vi "sub_thresh_swing_subvi.vi"(0 "Path":path, 9 "NumPts":dbl=3.0, 11 "Row Start":dbl=20.0) -> (3 "Index":dbl, 4 "XY Graph":cluster{dbl[], dbl[]}[](graph), 12 "Table Control":string[][](table), 13 "Table Control 2":string[][](table), 15 "Sub Threshold Swing":dbl)   [LabVIEW 2011]
uses:
  <vilib>/Utility/file.llb/Read From Spreadsheet File (string).vi
  <vilib>/Analysis/NI_AALPro.lvlib
panel:
  out "Numeric":dbl
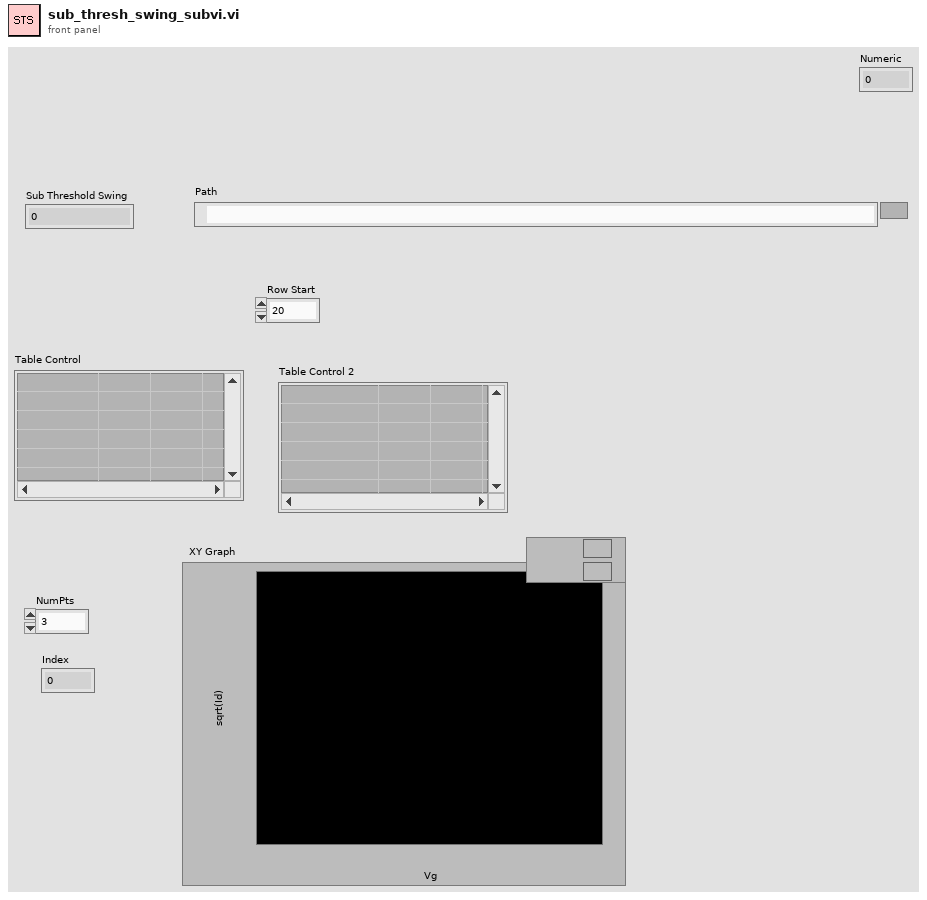
[diagram p1: front panel]
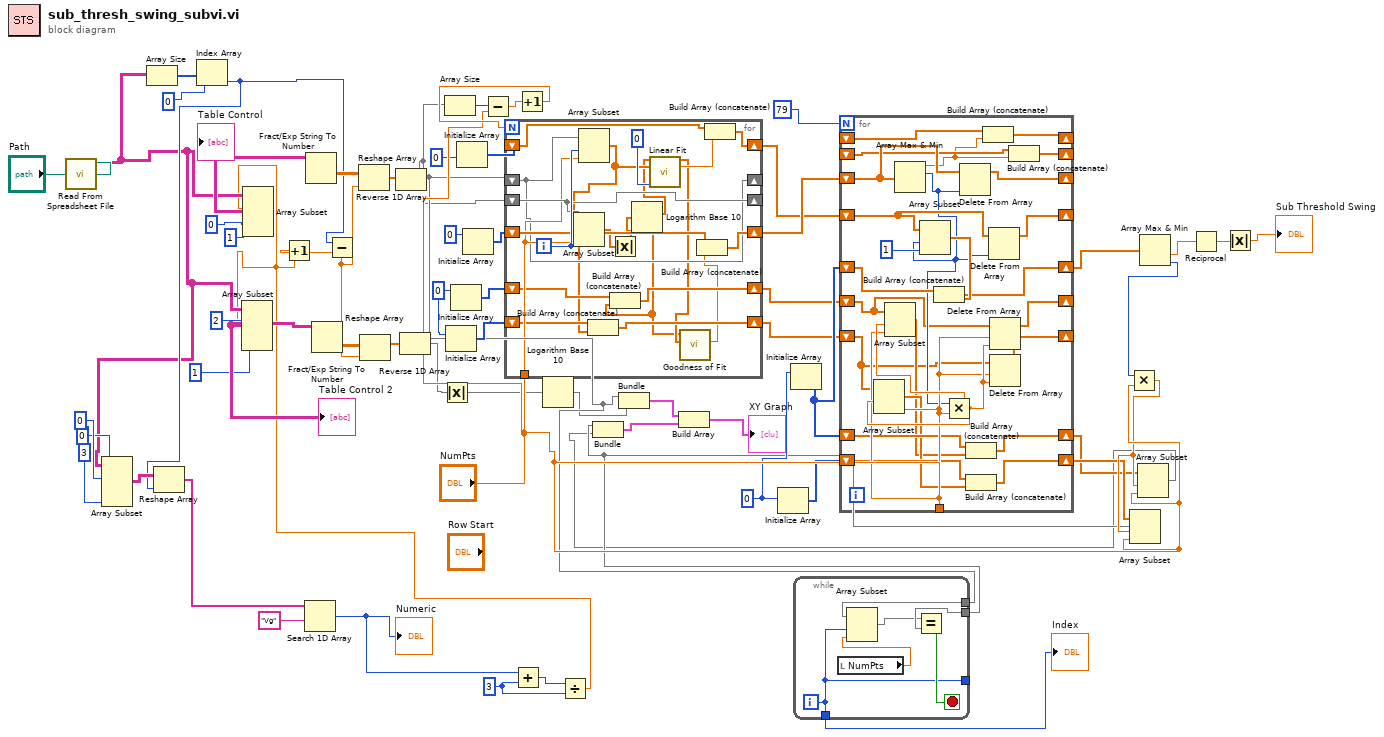
[diagram p0: block diagram]
diagram:
  w12 = 3
  w53 = 0
  w45 = 0
  n1 = call-poly <vilib>:"Read From Spreadsheet File.vi"("file path (dialog if empty)"="Path") -> ("all rows"=w3:string[][])  [unwired: 6 in, 4 out]
  n2 = Array Subset(array=w3, index (row)=0, index (col)=0, length (col)=3) -> (w5:string[][])  [unwired: 1 in]
  n3 = Array Size(array=w3) -> (size(s)=w41:i32[])
  n4 = Index Array(array=w41, index=0) -> (element=w4:i32)
  n5 = Reshape Array(w5, w4) -> (w2:string[])
  n6 = Search 1D Array(1D array=w2, element="Vg") -> (index of element=w10:i32)  [unwired: 1 in]
  "Numeric" <- w10
  n7 = Initialize Array(w45) -> (w47:i32[])  [unwired: 1 in]
  n8 = Initialize Array(w45) -> (w46:i32[])  [unwired: 1 in]
  n9 = Initialize Array(0) -> (w29:i32[])  [unwired: 1 in]
  n10 = Initialize Array(0) -> (w30:i32[])  [unwired: 1 in]
  n11 = Add(x=w10, y=w12) -> (x+y=w11:i32)
  n12 = Divide(x=w11, y=w12) -> (x/y=w1:dbl)
  n13 = Array Subset(array=w3, index (row)=w1, index (col)=2, length (col)=1) -> (w34:string[][])  [unwired: 1 in]
  "Table Control 2" <- w34
  n14 = Array Subset(array=w3, index (row)=w1, index (col)=0, length (col)=1) -> (w33:string[][])  [unwired: 1 in]
  "Table Control" <- w33
  n15 = Increment(x=w1) -> (x+1=w60:dbl)
  n16 = Fract/Exp String To Number(string=w33) -> (number=w35:dbl[][])  [unwired: 3 in, 1 out]
  n17 = Fract/Exp String To Number(string=w34) -> (number=w36:dbl[][])  [unwired: 3 in, 1 out]
  n18 = Subtract(x=w4, y=w60) -> (x-y=w61:dbl)
  n19 = Reshape Array(w35, w61) -> (w50:dbl[])
  n20 = Reshape Array(w36, w61) -> (w51:dbl[])
  n21 = Reverse 1D Array(array=w50) -> (reversed array=w22:dbl[])
  n22 = Reverse 1D Array(array=w51) -> (reversed array=w18:dbl[])
  n23 = Absolute Value(x=w18) -> (abs(x)=w17:dbl[])
  n24 = Array Size(array=w22) -> (size(s)=w28:i32)
  n25 = Subtract(x=w28, y="NumPts") -> (x-y=w63:dbl)
  n26 = Increment(x=w63) -> (x+1=w64:dbl)
  n27 = for {
    N: w64 -> [_]
    shift-right: [w71] -> _
    shift-left: w22 -> [w71]
    shift-right: [w78] -> _
    shift-left: w18 -> [w78]
    shift-right: [w82] -> w38
    shift-left: w29 -> [w81]
    shift-right: [w80] -> w42
    shift-left: w30 -> [w79]
    tunnel: "NumPts" -> [w76]
    shift-right: [w74] -> w48
    shift-left: w46 -> [w75]
    shift-right: [w72] -> w49
    shift-left: w47 -> [w73]
    i -> [w84]
    n28 = Array Subset(array=w78, index=w84, length=w76) -> (w65:dbl[])
    n29 = Array Subset(array=w71, index=w84, length=w76) -> (w70:dbl[])
    n30 = Build Array (concatenate)(w73, w70) -> (w72:dbl[])
    n31 = Absolute Value(x=w65) -> (abs(x)=w66:dbl[])
    n32 = Logarithm Base 10(1:w66) -> (0:w67:dbl[])
    n33 = Build Array (concatenate)(w75, w67) -> (w74:dbl[])
    n34 = call <vilib>:"Linear Fit.vi"("Y"=w67, "X"=w70, "method"=0) -> ("Best Linear Fit"=w69:dbl[], "slope"=w83:dbl)  [unwired: 8 in, 3 out]
    n35 = call <vilib>:"Goodness of Fit.vi"("Best Fit"=w69, "Y"=w67) -> ("R-square"=w68:dbl)  [unwired: 6 in, 3 out]
    n36 = Build Array (concatenate)(w79, w68) -> (w80:dbl[])
    n37 = Build Array (concatenate)(w81, w83) -> (w82:dbl[])
  }
  n38 = Logarithm Base 10(1:w17) -> (0:w19:dbl[])
  n39 = Bundle(w22, w19) -> (w44:cluster{dbl[], dbl[]})  [unwired: 1 in]
  n40 = Initialize Array(w53) -> (w52:i32[])  [unwired: 1 in]
  n41 = Initialize Array(w53) -> (w57:i32[])  [unwired: 1 in]
  n42 = for {
    N: 79 -> [_]
    shift-right: [w109] -> _
    shift-left: w42 -> [w110]
    shift-right: [w89] -> _
    shift-left: w38 -> [w90]
    shift-right: [w106] -> w39
    shift-left: w57 -> [w105]
    shift-right: [w104] -> _
    shift-left: _ -> [w103]
    shift-right: [w102] -> _
    shift-left: _ -> [w101]
    shift-right: [w100] -> _
    shift-left: w48 -> [w86]
    shift-right: [w98] -> _
    shift-left: w49 -> [w85]
    tunnel: "NumPts" -> [w97]
    shift-right: [w96] -> w54
    shift-left: w57 -> [w95]
    shift-right: [w94] -> w55
    shift-left: w52 -> [w93]
    n43 = Array Max & Min(array=w110) -> (max value=w88:dbl, max index (indices)=w87:i32)  [unwired: 2 out]
    n44 = Array Subset(array=w90, index=w87, length=1) -> (w107:dbl[])
    n45 = Build Array (concatenate)(w105, w107) -> (w106:dbl[])
    n46 = Multiply(x=w87, y=w97) -> (x*y=w99:dbl)
    n47 = Array Subset(array=w85, index=w99, length=w97) -> (w92:dbl[])
    n48 = Array Subset(array=w86, index=w99, length=w97) -> (w91:dbl[])
    n49 = Delete From Array(array=w110, index=w87) -> (array with subset deleted=w109:dbl[])  [unwired: 1 in, 1 out]
    n50 = Build Array (concatenate)(w95, w91) -> (w96:dbl[])
    n51 = Build Array (concatenate)(w93, w92) -> (w94:dbl[])
    n52 = Build Array (concatenate)(w103, w88) -> (w104:dbl[])
    n53 = Delete From Array(array=w90, index=w87) -> (array with subset deleted=w89:dbl[])  [unwired: 1 in, 1 out]
    n54 = Delete From Array(array=w86, length=w97, index=w99) -> (array with subset deleted=w100:dbl[])  [unwired: 1 out]
    n55 = Delete From Array(array=w85, length=w97, index=w99) -> (array with subset deleted=w98:dbl[])  [unwired: 1 out]
    n56 = Build Array (concatenate)(w101, w88) -> (w102:dbl[])
  }
  n57 = Array Max & Min(array=w39) -> (min value=w16:dbl, min index (indices)=w56:i32)  [unwired: 2 out]
  n58 = Multiply(x=w56, y="NumPts") -> (x*y=w58:dbl)
  n59 = Array Subset(array=w55, index=w58, length="NumPts") -> (w20:dbl[])
  n60 = while {
    tunnel: [w111] -> _
    tunnel: w22 -> [w115]
    tunnel: w20 -> [w114]
    tunnel: [w111] -> w21
    i -> [w111]
    stop <- w116 stop-if-true
    n61 = local read "NumPts"() -> (w112:dbl)
    n62 = Array Subset(array=w115, index=w111, length=w112) -> (w113:dbl[])
    n63 = Equal?(x=w113, y=w114) -> (x = y?=w116:bool)
  }
  "Index" <- w21
  n64 = Array Subset(array=w54, index=w58, length="NumPts") -> (w13:dbl[])
  n65 = Bundle(w20, w13) -> (w59:cluster{dbl[], dbl[]})  [unwired: 1 in]
  n66 = Build Array(w44, w59) -> (→"XY Graph":cluster{dbl[], dbl[]}[])
  n67 = Reciprocal(x=w16) -> (1/x=w15:dbl)
  n68 = Absolute Value(x=w15) -> (abs(x)=→"Sub Threshold Swing":dbl)
